vi "build_graph-multiple_axis.vi"(8 "error in (no error)":errorcluster, 10 "y_axis":cluster{dbl[][]}[](array[cluster]), 11 "x_axis":cluster{dbl[]}[](array[cluster])) -> (0 "error out":errorcluster, 4 "graph_data":cluster{dbl[], dbl[]}[](array[cluster]), 6 "scale_range":T1)   [LabVIEW 2015, in "lv-graph.lvlib"]
uses:
  lv-graph.lvlib
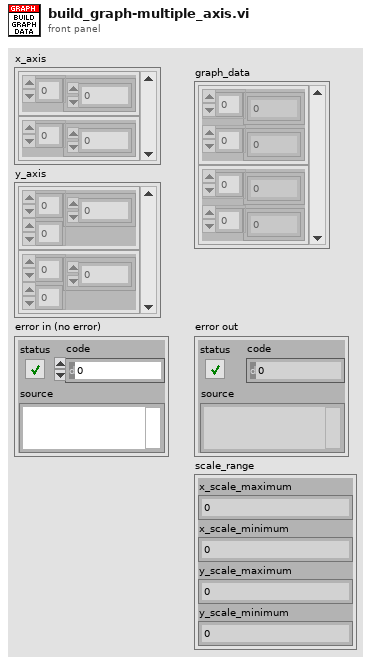
[diagram p1: front panel]
types:
  T1 = cluster{"x_scale_maximum":dbl, "x_scale_minimum":dbl, "y_scale_maximum":dbl, "y_scale_minimum":dbl}
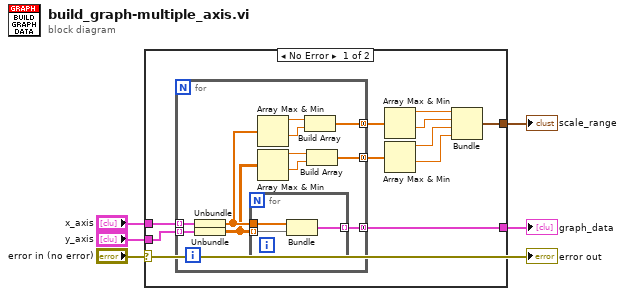
[diagram p0: block diagram]
diagram:
  n1 = case shown="No Error" "error in (no error)" {
    tunnel: [w15 _] -> w5
    tunnel: "y_axis" -> [w14 _]
    tunnel: "x_axis" -> [w13 _]
    tunnel: [w12 _] -> w3
    frame No Error {
      n2 = for {
        tunnel: w13 -> [w26] mode=indexing
        tunnel: w14 -> [w24] mode=indexing
        tunnel: [w25] -> w15 mode=concatenating
        tunnel: [w17] -> w10 mode=concatenating
        tunnel: [w16] -> w11 mode=concatenating
        n3 = Unbundle(w26) -> (w23:dbl[])
        n4 = Unbundle(w24) -> (w22:dbl[][])
        n5 = for {
          tunnel: [w29] -> w25 mode=indexing
          tunnel: w22 -> [w28] mode=indexing
          tunnel: w23 -> [w27]
          n6 = Bundle(w27, w28) -> (w29:cluster{dbl[], dbl[]})  [unwired: 1 in]
        }
        n7 = Array Max & Min(array=w23) -> (max value=w21:dbl, min value=w20:dbl)  [unwired: 2 out]
        n8 = Array Max & Min(array=w22) -> (max value=w19:dbl, min value=w18:dbl)  [unwired: 2 out]
        n9 = Build Array(w21, w20) -> (w16:dbl[])
        n10 = Build Array(w19, w18) -> (w17:dbl[])
      }
      n11 = Array Max & Min(array=w11) -> (max value=w9:dbl, min value=w8:dbl)  [unwired: 2 out]
      n12 = Array Max & Min(array=w10) -> (max value=w7:dbl, min value=w6:dbl)  [unwired: 2 out]
      n13 = Bundle(w9, w8, w7, w6) -> (w12:cluster{dbl, dbl, dbl, dbl})  [unwired: 1 in]
    }
    frame Error {
    }
  }
  "graph_data" <- w5
  "scale_range" <- w3
  "error out" <- "error in (no error)"
